vi "Get Item by name.vi"(8 "error in (no error)":errorcluster, 10 "name":string, 11 "JSON Array In":refnum<class "JSON Array.lvclass">) -> (0 "error out":errorcluster, 1 "found":bool, 2 "Value":refnum<class "JSON Value.lvclass">, 3 "JSON Array Out":refnum<class "JSON Array.lvclass">)   [LabVIEW 2011, in "JSON Array.lvclass"]
uses:
  JSON Array.lvclass
  JSON Value/JSON Value.lvclass
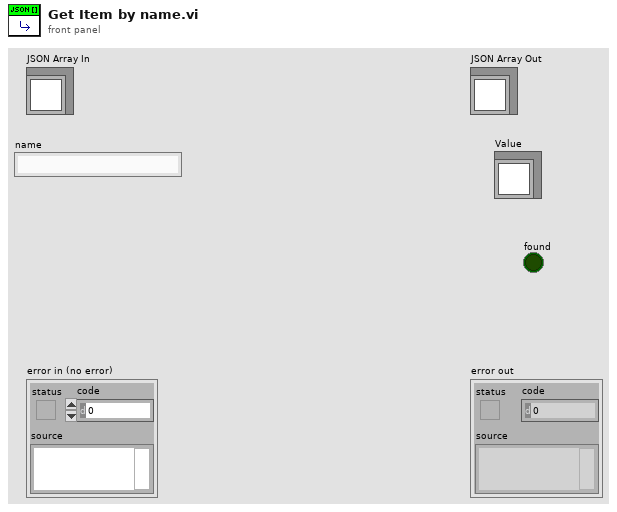
[diagram p1: front panel]
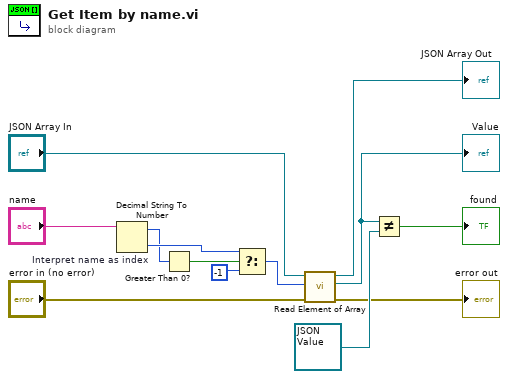
[diagram p0: block diagram]
diagram:
  n1 = Decimal String To Number "Interpret name as index"(string="name") -> (offset past number=w10:i32, number=w12:i32)  [unwired: 2 in]
  n2 = Greater Than 0?(x=w10) -> (x > 0?=w11:bool)
  n3 = Select(t=w12, s=w11, f=-1) -> (s? t:f=w1:i32)
  n4 = call "Read Element of Array.vi"("error in (no error)"="error in (no error)", "index"=w1, "JSON Array in"="JSON Array In") -> ("error out"=→"error out":errorcluster, "JSON Value.lvclass"=w4:refnum<class "JSON Value.lvclass">, "JSON Array out"=→"JSON Array Out":refnum<class "JSON Array.lvclass">)  [unwired: 6 in]
  "Value" <- w4
  n5 = Not Equal?(x=w4, y=refnum<class "JSON Value.lvclass"> refnum ("JSON Value.lvclass")) -> (x != y?=→"found":bool)
